vi "Teleop.vi"(10 "Match Info":T1={"Autonomous Elapsed Seconds"=0.0, "TeleOp Elapsed Seconds"=0.0, "Disabled Elapsed Seconds"=0.0, "Visited Autonomous"=FALSE, "Visited TeleOp"=FALSE, "Visited Disabled"=FALSE, "Autonomous Settings"={"Autonomous Style"=enum."Independent", "VI Refnum"=refnum}}, 11 "Call Context":T2) -> ()   [LabVIEW 2017]
doc: "This VI is called for each TeleOp packet received from the DS where the robot is not disabled. It is often used to read from the joysticks and update I/O or to update setpoints for timed control loops. It should complete and return within 20 milliseconds or it may miss DS packets."
uses:
  <vilib>/Rock Robotics/WPI/DriverStation/WPI_DriverStationDerivedRobotMode.ctl
  <vilib>/Rock Robotics/WPI/DriverStation/WPI_DriverStationMatch Info.ctl
  Lift States.ctl
  Robot Global Data.vi
  Joystick Values.vi
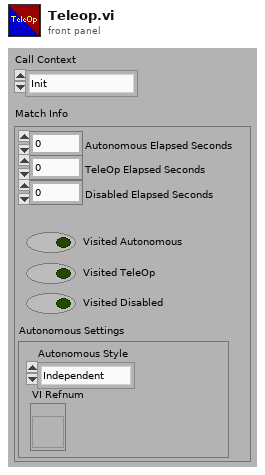
[diagram p1: front panel]
types:
  T1 = typedef "WPI_DriverStationMatch Info.ctl" = cluster{"Autonomous Elapsed Seconds":dbl, "TeleOp Elapsed Seconds":dbl, "Disabled Elapsed Seconds":dbl, "Visited Autonomous":bool, "Visited TeleOp":bool, "Visited Disabled":bool, "Autonomous Settings":cluster{"Autonomous Style":enum16{"Iterative", "Independent"}, "VI Refnum":refnum<vi>}}
  T2 = typedef "WPI_DriverStationDerivedRobotMode.ctl" = enum16{"Init", "Execute", "Stop"}
  T3 = typedef "Lift States.ctl" = enum16{"Manual", "Scale Low", "Scale Middle", "Scale High", "Rock Bottom", "Almost Down"}
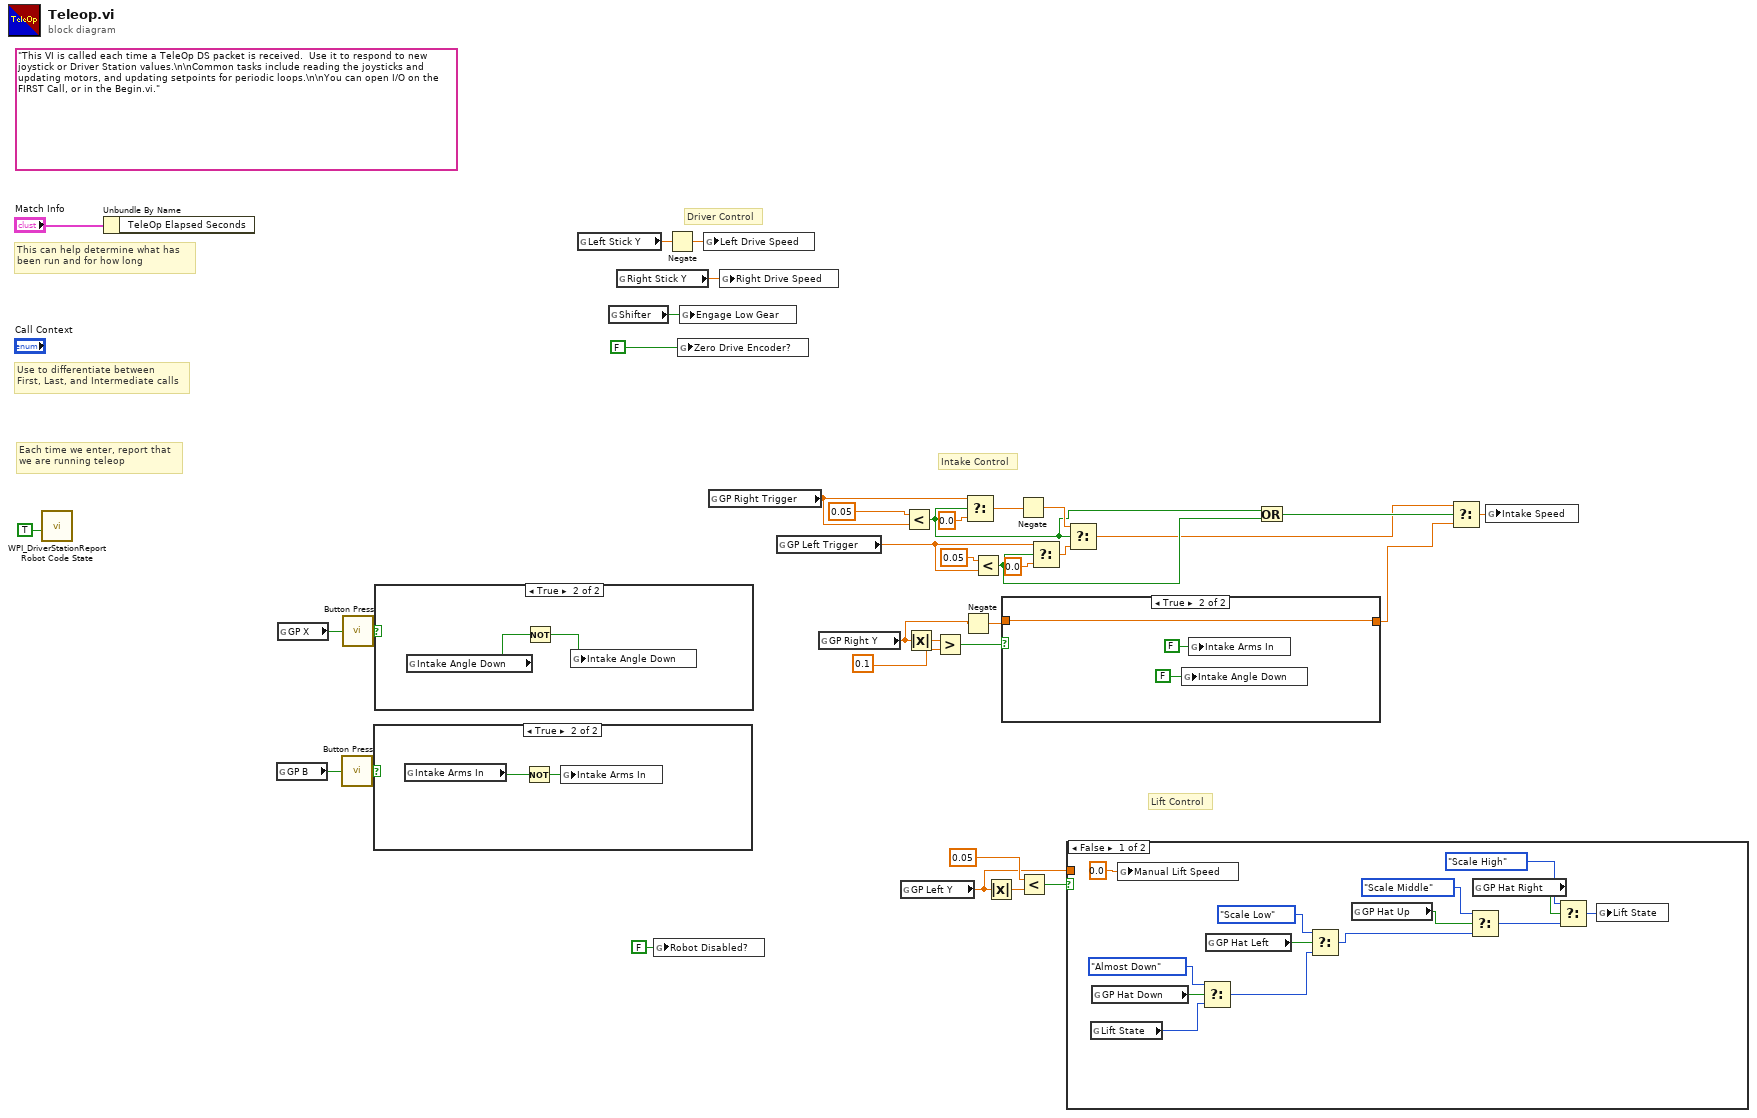
[diagram p0: block diagram]
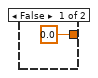
[diagram p2: hidden frame]
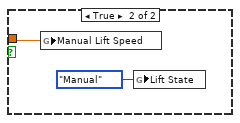
[diagram p5: hidden frame]
diagram:
  (unwired) "This VI is called each time a TeleOp DS packet is received.  Use it to respond to new joystick or Driver Station values.\n\nCommon tasks include reading the joysticks and updating motors, and updating setpoints for periodic loops.\n\nYou can open I/O on the FIRST Call, or in the Begin.vi."
  # "Driver Control"
  # "Intake Control"
  # "Lift Control"
  # "Each time we enter, report that\nwe are running teleop"
  # "Use to differentiate between\nFirst, Last, and Intermediate calls"
  # "This can help determine what has\nbeen run and for how long"
  n1 = call <vilib>:"WPI_DriverStationReport Robot Code State.vi"("TeleOp"=TRUE ("Autonomous")) -> ()  [unwired: 10 in, 1 out]
  n2 = Unbundle By Name("Match Info") -> ()  [unwired: 1 out]
  n3 = global read "Joystick Values.vi" "GP B"() -> (w18:bool)
  n4 = global read "Joystick Values.vi" "GP X"() -> (w21:bool)
  n5 = call "Button Press.vi"("Current Button"=w18) -> ("Pressed?"=w17:bool)
  n6 = call "Button Press.vi"("Current Button"=w21) -> ("Pressed?"=w20:bool)
  n7 = case shown="True" w17 {
    frame False {
    }
    frame True {
      n8 = global read "Robot Global Data.vi" "Intake Arms In"() -> (w38:bool)
      n9 = Not(x=w38) -> (.not. x?=w37:bool)
      n10 = global write "Robot Global Data.vi" "Intake Arms In"(w37) -> ()
    }
  }
  n11 = case shown="True" w20 {
    frame False {
    }
    frame True {
      n12 = global read "Robot Global Data.vi" "Intake Angle Down"() -> (w40:bool)
      n13 = Not(x=w40) -> (.not. x?=w39:bool)
      n14 = global write "Robot Global Data.vi" "Intake Angle Down"(w39) -> ()
    }
  }
  n15 = global read "Joystick Values.vi" "Left Stick Y"() -> (w6:dbl)
  n16 = global read "Joystick Values.vi" "Shifter"() -> (w4:bool)
  n17 = global read "Joystick Values.vi" "Right Stick Y"() -> (w7:dbl)
  n18 = global write "Robot Global Data.vi" "Robot Disabled?"(FALSE ("AUTO Start Left")) -> ()
  n19 = Negate(x=w6) -> (-x=w5:dbl)
  n20 = global write "Robot Global Data.vi" "Zero Drive Encoder?"(FALSE ("Zero Drive Encoder?")) -> ()
  n21 = global write "Robot Global Data.vi" "Engage Low Gear"(w4) -> ()
  n22 = global write "Robot Global Data.vi" "Left Drive Speed"(w5) -> ()
  n23 = global read "Joystick Values.vi" "GP Right Trigger"() -> (w29:dbl)
  n24 = global write "Robot Global Data.vi" "Right Drive Speed"(w7) -> ()
  n25 = global read "Joystick Values.vi" "GP Left Trigger"() -> (w24:dbl)
  n26 = global read "Joystick Values.vi" "GP Right Y"() -> (w3:dbl)
  n27 = global read "Joystick Values.vi" "GP Left Y"() -> (w31:dbl)
  n28 = Less?(x=0.05, y=w29) -> (x < y?=w15:bool)
  n29 = Absolute Value(x=w3) -> (abs(x)=w10:dbl)
  n30 = Greater?(x=w10, y=0.1) -> (0:w9:bool)
  n31 = Negate(x=w3) -> (-x=w2:dbl)
  n32 = Select(t=w29, s=w15, f=0.0) -> (s? t:f=w27:dbl)
  n33 = Less?(x=0.05, y=w24) -> (x < y?=w16:bool)
  n34 = Absolute Value(x=w31) -> (abs(x)=w34:dbl)
  n35 = case shown="True" w9 {
    tunnel: [0.0 ("y") w42] -> w12
    tunnel: w2 -> [_ w42]
    frame False {
    }
    frame True {
      n36 = global write "Robot Global Data.vi" "Intake Angle Down"(FALSE ("Intake Arms In")) -> ()
      n37 = global write "Robot Global Data.vi" "Intake Arms In"(FALSE ("Intake Arms In")) -> ()
    }
  }
  n38 = Negate(x=w27) -> (-x=w22:dbl)
  n39 = Less?(x=0.05, y=w34) -> (x < y?=w32:bool)
  n40 = Select(t=w24, s=w16, f=0.0) -> (s? t:f=w23:dbl)
  n41 = case shown="False" w32 {
    tunnel: w31 -> [_ w59]
    frame False {
      n42 = global read "Robot Global Data.vi" "Lift State"() -> (w55:T3)
      n43 = global read "Joystick Values.vi" "GP Hat Down"() -> (w57:bool)
      n44 = global write "Robot Global Data.vi" "Manual Lift Speed"(0.0 ("Lift Speed")) -> ()
      n45 = Select(t=Lift_States."Almost Down" ("Lift State"), s=w57, f=w55) -> (s? t:f=w45:T3)
      n46 = global read "Joystick Values.vi" "GP Hat Left"() -> (w48:bool)
      n47 = Select(t=Lift_States."Scale Low" ("Lift State"), s=w48, f=w45) -> (s? t:f=w46:T3)
      n48 = global read "Joystick Values.vi" "GP Hat Up"() -> (w54:bool)
      n49 = Select(t=Lift_States."Scale Middle" ("Lift State"), s=w54, f=w46) -> (s? t:f=w52:T3)
      n50 = global read "Joystick Values.vi" "GP Hat Right"() -> (w53:bool)
      n51 = Select(t=Lift_States."Scale High" ("Lift State"), s=w53, f=w52) -> (s? t:f=w49:T3)
      n52 = global write "Robot Global Data.vi" "Lift State"(w49) -> ()
    }
    frame True {
      n53 = global write "Robot Global Data.vi" "Manual Lift Speed"(w59) -> ()
      n54 = global write "Robot Global Data.vi" "Lift State"(Lift_States."Manual" ("Lift State")) -> ()
    }
  }
  n55 = Select(t=w22, s=w15, f=w23) -> (s? t:f=w13:dbl)
  n56 = Or(x=w15, y=w16) -> (x .or. y?=w14:bool)
  n57 = Select(t=w13, s=w14, f=w12) -> (s? t:f=w11:dbl)
  n58 = global write "Robot Global Data.vi" "Intake Speed"(w11) -> ()
